vi "Sensor HW Read.vi"(8 "Error":errorcluster, 9 "Read Closed Loop":bool, 11 "Ref":T7) -> (0 "Error Out":errorcluster, 2 "Sensor Values Out":T1, 3 "DevRef Out":T7)   [LabVIEW 2023, in "Pivot FX_ACT.lvlib"]
uses:
  Pivot FX_ACT.lvlib
  Shared Code/TypeDefs/Cluster_FX CloseLoop Values.ctl
  Shared Code/TypeDefs/Cluster_FX Current Values.ctl
  Cluster_HW Output Values.ctl
  Shared Code/TypeDefs/Cluster_FX Limit Switchs.ctl
  Shared Code/TypeDefs/Cluster_FX Voltage Values.ctl
  Shared Code/TypeDefs/Cluster_FX Sensor Values.ctl
  <vilib>/Rock Robotics/SystemInterfaces/DIO/FPGA_DIOPWMChannel.ctl
  <vilib>/Rock Robotics/WPI/PWM/WPI_PWMDeadband.ctl
  <vilib>/Rock Robotics/WPI/MotorControl/WPI_MotorControlType.ctl
  <vilib>/Rock Robotics/SystemInterfaces/DIO/FPGA_DIOChannel.ctl
  <vilib>/Rock Robotics/WPI/MotorControl/WPI_MotorControlDeviceRef.ctl
panel:
  in  "CL Slot":i32
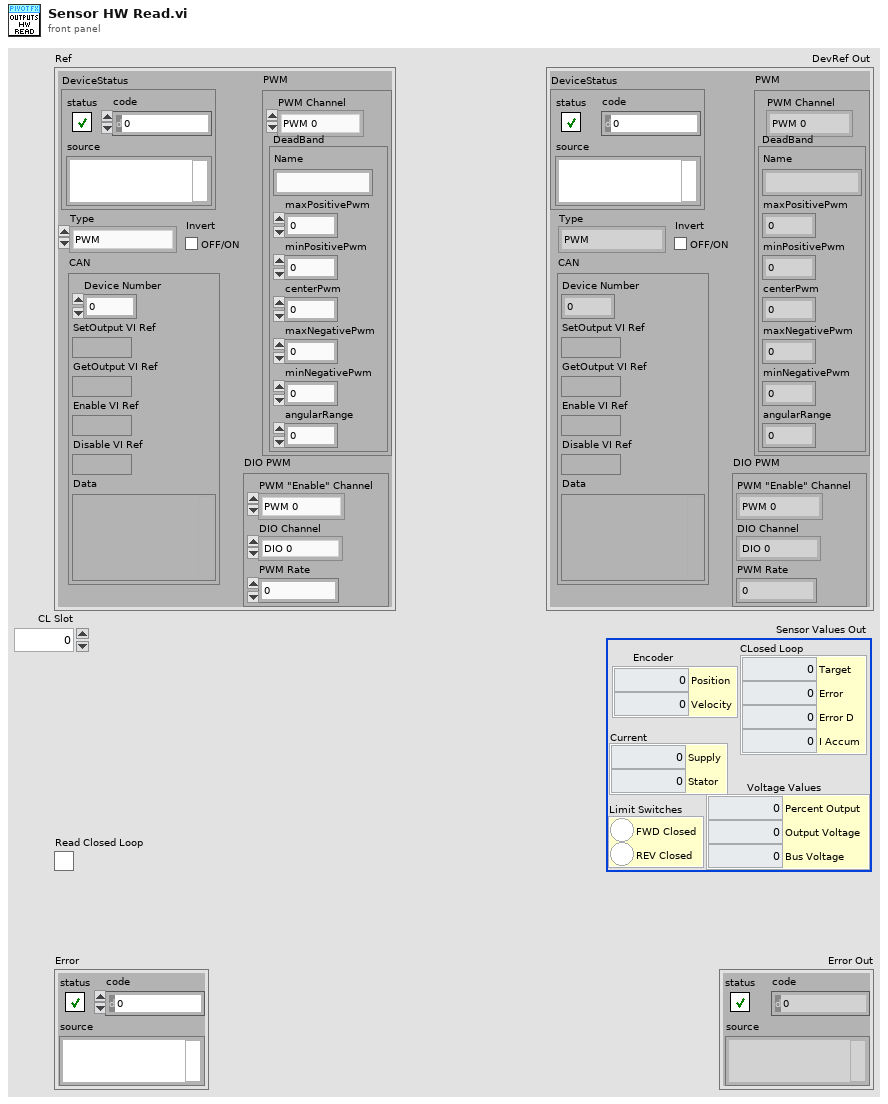
[diagram p1: front panel]
types:
  T1 = typedef "Pivot FX_ACT.lvlib/Cluster_HW Output Values.ctl" = cluster{"CLosed Loop":T2, "Current":T3, "Limit Switches":T4, "Voltage Values":T5, "Encoder ":T6}
  T2 = typedef "Cluster_FX CloseLoop Values.ctl" = cluster{"Target":dbl, "Error":i32, "Error D":dbl, "I Accum":dbl}
  T3 = typedef "Cluster_FX Current Values.ctl" = cluster{"Supply":dbl, "Stator":dbl}
  T4 = typedef "Cluster_FX Limit Switchs.ctl" = cluster{"FWD Closed":bool, "REV Closed":bool}
  T5 = typedef "Cluster_FX Voltage Values.ctl" = cluster{"Percent Output":dbl, "Output Voltage":dbl, "Bus Voltage":dbl}
  T6 = typedef "Cluster_FX Sensor Values.ctl" = cluster{"Position":i32, "Velocity":i32}
  T7 = typedef "WPI_MotorControlDeviceRef.ctl" = cluster{"DeviceStatus":errorcluster, "Type":T8, "PWM":cluster{"PWM Channel":T9, "DeadBand":T10}, "CAN":cluster{"Device Number":u8, "SetOutput VI Ref":variant, "GetOutput VI Ref":variant, "Enable VI Ref":variant, "Disable VI Ref":variant, "Data":variant}, "Invert":bool, "DIO PWM":cluster{"PWM \"Enable\" Channel":T9, "DIOChannel":T11, "PWM Rate":dbl}}
  T8 = typedef "WPI_MotorControlType.ctl" = enum16{"PWM", "CAN", "DIO PWM"}
  T9 = typedef "FPGA_DIOPWMChannel.ctl" = enum8{"PWM 0", "PWM 1", "PWM 2", "PWM 3", "PWM 4", "PWM 5", "PWM 6", "PWM 7", "PWM 8", "PWM 9", "PWM MXP 0", "PWM MXP 1", "PWM MXP 2", "PWM MXP 3", "PWM MXP 4", "PWM MXP 5", "PWM MXP 6", "PWM MXP 7", "PWM MXP 8", "PWM MXP 9", "Invalid"}
  T10 = typedef "WPI_PWMDeadband.ctl" = cluster{"Name":string, "maxPositivePwm":i32, "minPositivePwm":i32, "centerPwm":i32, "maxNegativePwm":i32, "minNegativePwm":i32, "angularRange":u16}
  T11 = typedef "FPGA_DIOChannel.ctl" = enum8{"DIO 0", "DIO 1", "DIO 2", "DIO 3", "DIO 4", "DIO 5", "DIO 6", "DIO 7", "DIO 8", "DIO 9", "DIO MXP 0", "DIO MXP 1", "DIO MXP 2", "DIO MXP 3", "DIO MXP 4", "DIO MXP 5", "DIO MXP 6", "DIO MXP 7", "DIO MXP 8", "DIO MXP 9", "DIO MXP 10", "DIO MXP 11", "DIO MXP 12", "DIO MXP 13", "DIO MXP 14", "DIO MXP 15", "SPI Port CS1", "SPI Port CS2", "SPI Port CS3", "SPI Port MISO", "SPI Port MOSI", "Invalid"}
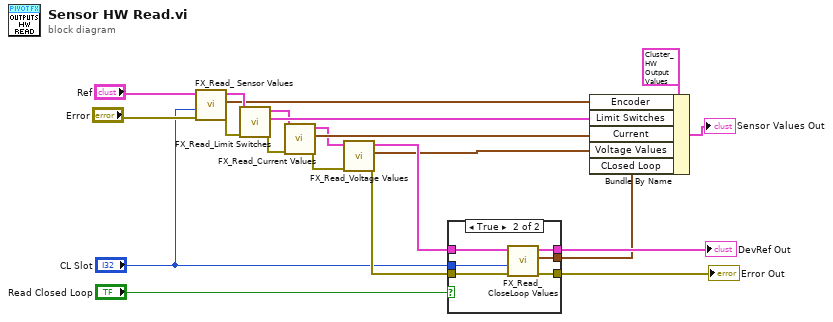
[diagram p0: block diagram]
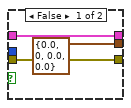
[diagram p2: hidden frame]
diagram:
  n1 = call "FX_Read_ Sensor Values.vi"("Error"="Error", "PidLoopIdx"="CL Slot", "PhoenixMotorControlDevRef"="Ref") -> ("Error Out"=w20:errorcluster, "Encoder Values Out"=w18:T6, "PhoenixMotorControlDevRef Out"=w21:T7)  [unwired: 6 in]
  n2 = call "FX_Read_Limit Switches.vi"("Error"=w20, "PhoenixMotorControlDevRef"=w21) -> ("Error Out"=w13:errorcluster, "Limit Switches Out"=w19:T4, "PhoenixMotorControlDevRef Out"=w16:T7)  [unwired: 7 in]
  n3 = call "FX_Read_Current Values.vi"("error in"=w13, "PhoenixMotorControlDevRef in"=w16) -> ("error out"=w4:errorcluster, "Current Values"=w17:T3, "PhoenixMotorControlDevRef out"=w6:T7)  [unwired: 7 in]
  n4 = call "FX_Read_Voltage Values.vi"("Error"=w4, "PhoenixMotorControlDevRef"=w6) -> ("Error Out"=w3:errorcluster, "Voltage Cluster Out"=w2:T5, "PhoenixMotorControlDevRef Out"=w5:T7)  [unwired: 7 in]
  n5 = case shown="True" "Read Closed Loop" {
    tunnel: w5 -> [w24 w30]
    tunnel: [w24 w29] -> w12
    tunnel: [T2 {"Target"=0.0, "Error"=0, "Error D"=0.0, "I Accum"=0.0} ("CLosed Loop Out") w28] -> w11
    tunnel: "CL Slot" -> [_ w25]
    tunnel: w3 -> [w22 w27]
    tunnel: [w22 w26] -> w9
    frame False {
    }
    frame True {
      n6 = call "FX_Read_CloseLoop Values.vi"("Error"=w27, "Slot"=w25, "PhoenixMotorControlDevRef"=w30) -> ("Error Out"=w26:errorcluster, "CLosed Loop Out"=w28:T2, "PhoenixMotorControlDevRef Out"=w29:T7)  [unwired: 6 in]
    }
  }
  "DevRef Out" <- w12
  "Error Out" <- w9
  n7 = Bundle By Name(cluster=T1 {"CLosed Loop"={"Target"=0.0, "Error"=0, "Error D"=0.0, "I Accum"=0.0}, "Current"={"Supply"=0.0, "Stator"=0.0}, "Limit Switches"={"FWD Closed"=FALSE, "REV Closed"=FALSE}, "Voltage Values"={"Percent Output"=0.0, "Output Voltage"=0.0, "Bus Voltage"=0.0}, "Encoder "={"Position"=0, "Velocity"=0}} ("Sensor Values Out"), "Encoder"=w18, "Limit Switches"=w19, "Current"=w17, "Voltage Values"=w2, "CLosed Loop"=w11) -> (→"Sensor Values Out":T1)
